vi "cluster_append.vi"(4 "Trigger line":i32, 6 "Rotary encoder":dbl, 8 "Input Cluster":T1={"Magnitude meas."=[], "Phase meas."=[], "Shift meas."=[], "cw"=TRUE, "projections per image"=0, "ramp-up readouts"=0, "current sense type"="", "Number of pulses per image"=0, "Rotation enabled"=TRUE, "Rotary position"=[], "Baseline magnitude"=0.0, "Baseline phase"=0.0, "Wait readouts"=0, "Shift waveform type"="", "Shift enabled"=TRUE, "Time domain data"=[], "Motor pulse duration"=0.0, "Shift start"=0.0, "Shift stop"=0.0, "Notes"="", "Reconstructed image"=bytes[0], "Rotary encoder type"="", "Image start"=timestamp(0 s since 1904-01-01), "Image stop"=timestamp(0 s since 1904-01-01), "readouts per projection"=0, "Recon enabled"=FALSE, "Bidirectional shift"=FALSE, "Imager mode"="", "Shift delay"=0.0, "Shift frequency"=0.0, "Image time (calc)"=0.0, "Initial encoder position"=0.0, "Recon data"=[], "Trigger line values"=[], "Bed position"=0.0, "Sample image"=bytes[0], "Patch amplitude"=0.0, "Patch frequency"=0.0, "Patch phase"=0.0}, 9 "shift value":dbl, 10 "phase value":dbl, 11 "magnitude value":dbl) -> (0 "Output Cluster":T1={"Magnitude meas."=[], "Phase meas."=[], "Shift meas."=[], "cw"=TRUE, "projections per image"=0, "ramp-up readouts"=0, "current sense type"="", "Number of pulses per image"=0, "Rotation enabled"=TRUE, "Rotary position"=[], "Baseline magnitude"=0.0, "Baseline phase"=0.0, "Wait readouts"=0, "Shift waveform type"="", "Shift enabled"=TRUE, "Time domain data"=[], "Motor pulse duration"=0.0, "Shift start"=0.0, "Shift stop"=0.0, "Notes"="", "Reconstructed image"=bytes[0], "Rotary encoder type"="", "Image start"=timestamp(0 s since 1904-01-01), "Image stop"=timestamp(0 s since 1904-01-01), "readouts per projection"=0, "Recon enabled"=FALSE, "Bidirectional shift"=FALSE, "Imager mode"="", "Shift delay"=0.0, "Shift frequency"=0.0, "Image time (calc)"=0.0, "Initial encoder position"=0.0, "Recon data"=[], "Trigger line values"=[], "Bed position"=0.0, "Sample image"=bytes[0], "Patch amplitude"=0.0, "Patch frequency"=0.0, "Patch phase"=0.0})   [LabVIEW 2019]
panel:
  # "Append Values to Cluster arrays"
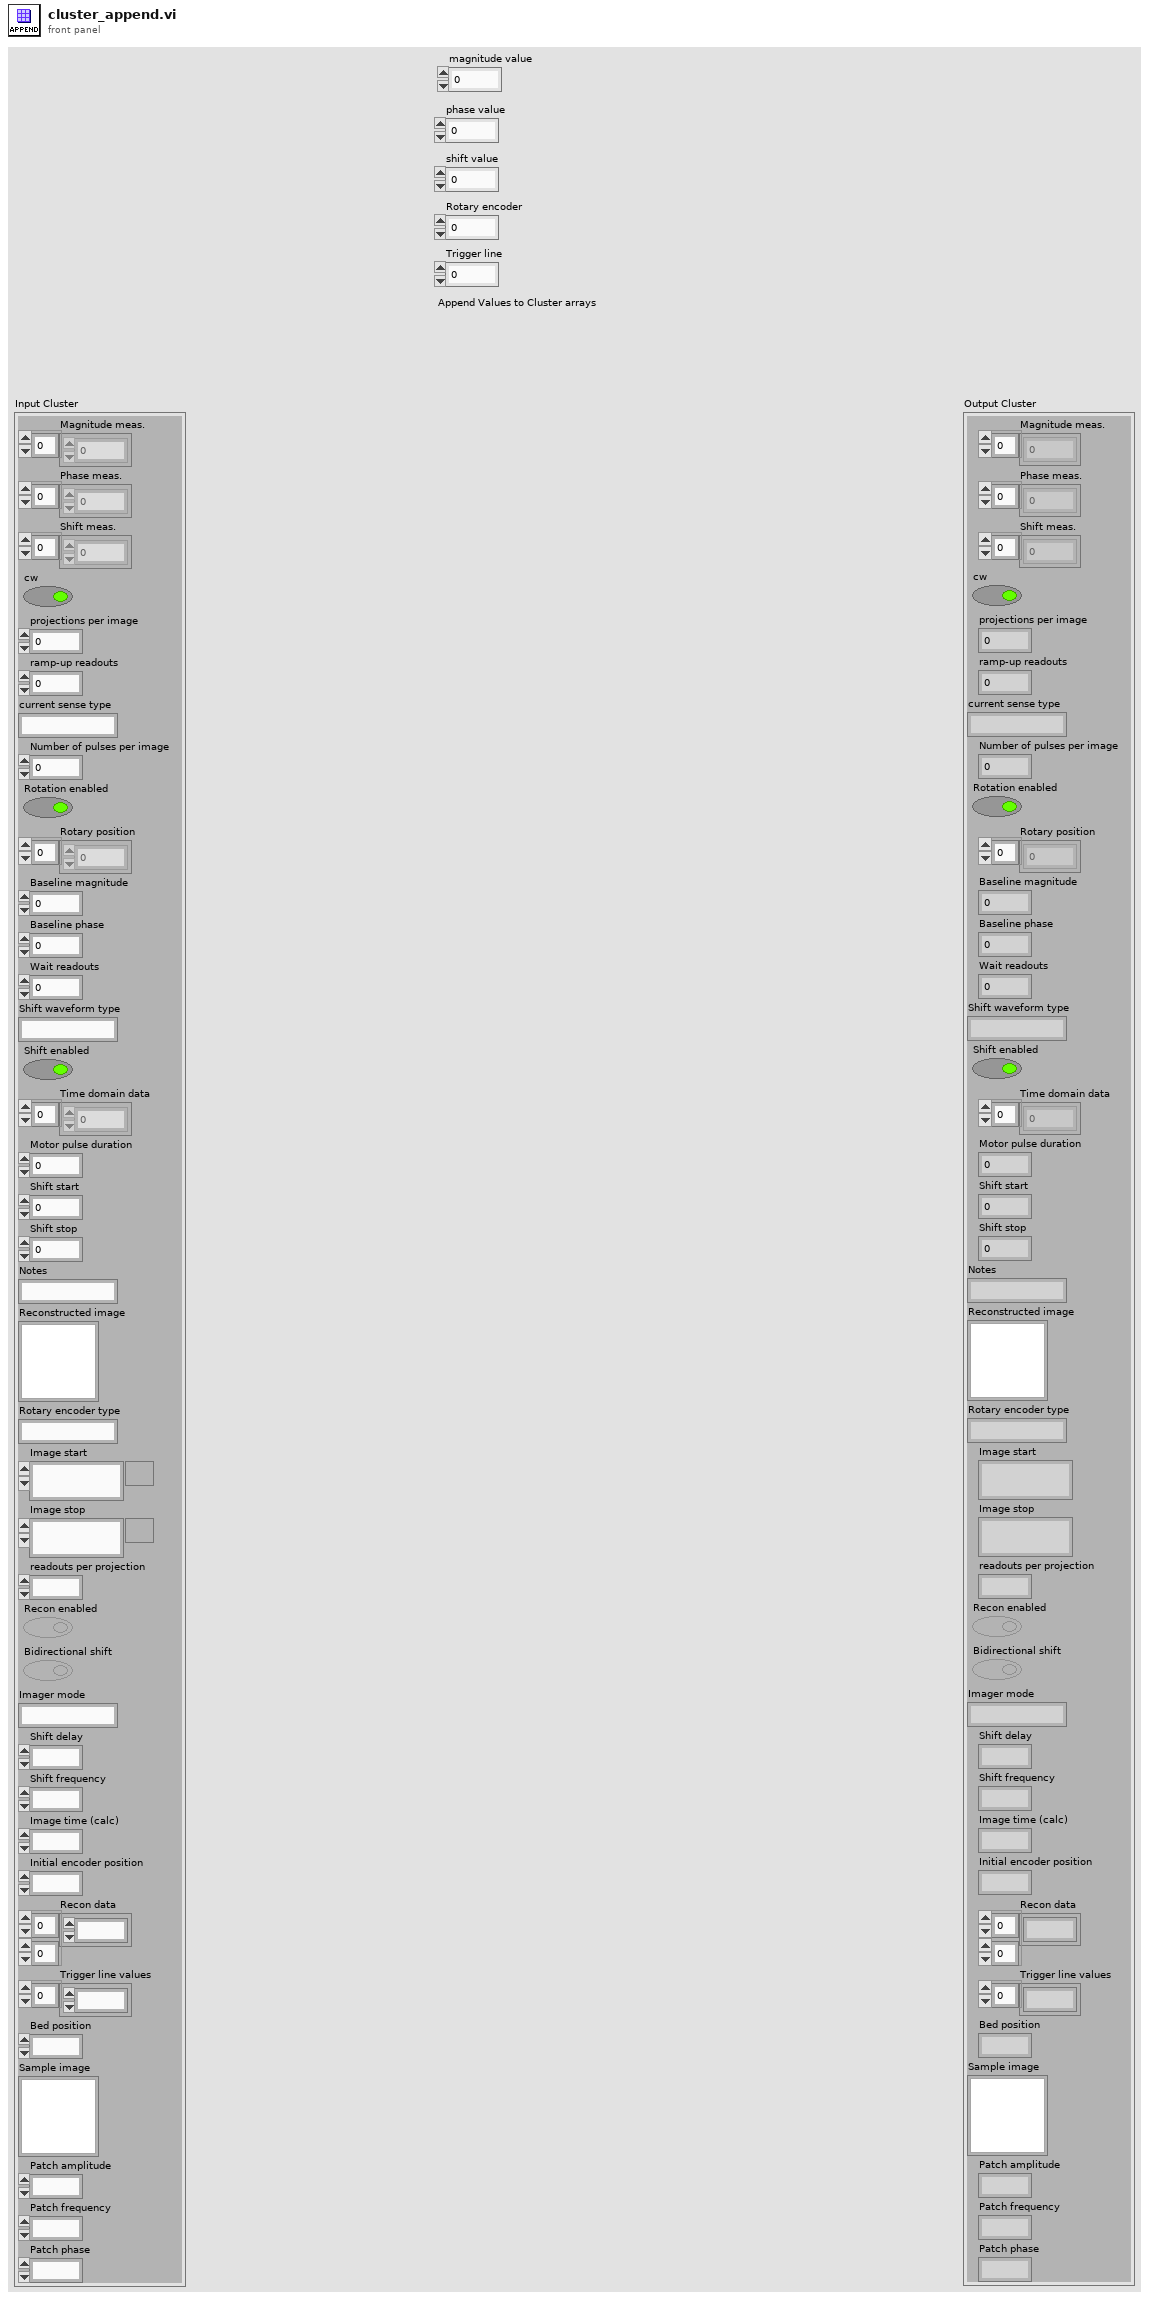
[diagram p1: front panel]
types:
  T1 = cluster{"Magnitude meas.":dbl[], "Phase meas.":dbl[], "Shift meas.":dbl[], "cw":bool, "projections per image":i32, "ramp-up readouts":i32, "current sense type":string, "Number of pulses per image":i32, "Rotation enabled":bool, "Rotary position":dbl[], "Baseline magnitude":dbl, "Baseline phase":dbl, "Wait readouts":i32, "Shift waveform type":string, "Shift enabled":bool, "Time domain data":dbl[], "Motor pulse duration":dbl, "Shift start":dbl, "Shift stop":dbl, "Notes":string, "Reconstructed image":picture, "Rotary encoder type":string, "Image start":timestamp, "Image stop":timestamp, "readouts per projection":i32, "Recon enabled":bool, "Bidirectional shift":bool, "Imager mode":string, "Shift delay":dbl, "Shift frequency":dbl, "Image time (calc)":dbl, "Initial encoder position":dbl, "Recon data":dbl[][], "Trigger line values":i32[], "Bed position":dbl, "Sample image":picture, "Patch amplitude":dbl, "Patch frequency":dbl, "Patch phase":dbl}
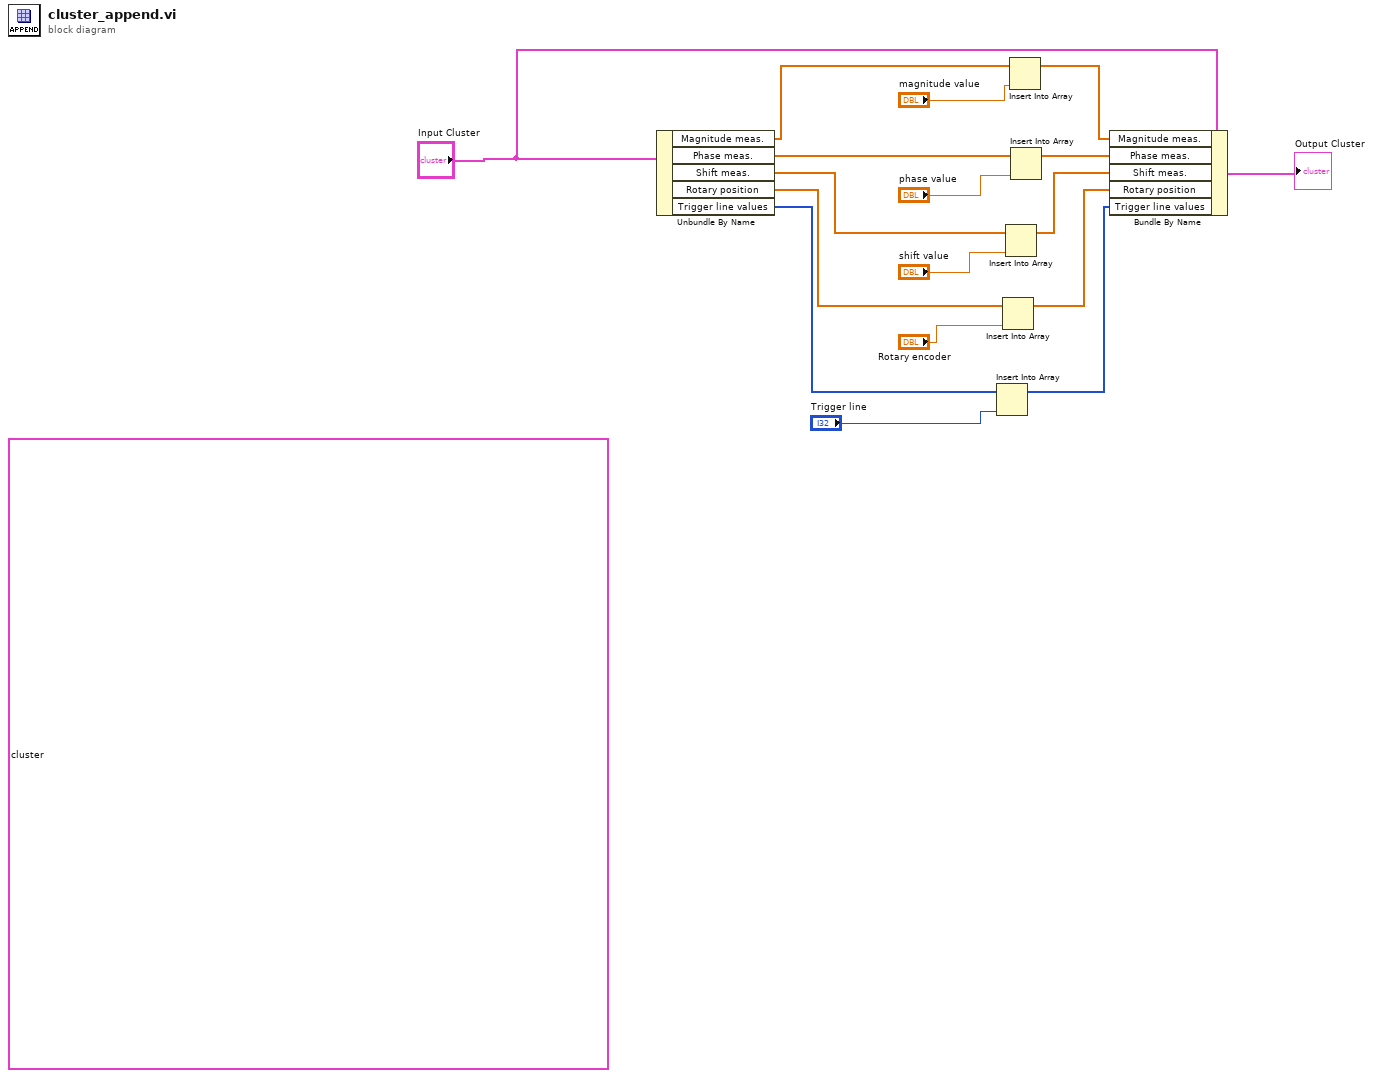
[diagram p0: block diagram]
diagram:
  (unwired) T1 {"Magnitude meas."=[], "Phase meas."=[], "Shift meas."=[], "cw"=TRUE, "projections per image"=0, "ramp-up readouts"=0, "current sense type"="", "Number of pulses per image"=0, "Rotation enabled"=TRUE, "Rotary position"=[], "Baseline magnitude"=0.0, "Baseline phase"=0.0, "Wait readouts"=0, "Shift waveform type"="", "Shift enabled"=TRUE, "Time domain data"=[], "Motor pulse duration"=0.0, "Shift start"=0.0, "Shift stop"=0.0, "Notes"="", "Reconstructed image"=bytes[0], "Rotary encoder type"="", "Image start"=timestamp(0 s since 1904-01-01), "Image stop"=timestamp(0 s since 1904-01-01), "readouts per projection"=0, "Recon enabled"=FALSE, "Bidirectional shift"=FALSE, "Imager mode"="", "Shift delay"=0.0, "Shift frequency"=0.0, "Image time (calc)"=0.0, "Initial encoder position"=0.0, "Recon data"=[], "Trigger line values"=[], "Bed position"=0.0, "Sample image"=bytes[0], "Patch amplitude"=0.0, "Patch frequency"=0.0, "Patch phase"=0.0}
  n1 = Unbundle By Name("Input Cluster") -> ("Magnitude meas."=w12:dbl[], "Phase meas."=w15:dbl[], "Shift meas."=w13:dbl[], "Rotary position"=w7:dbl[], "Trigger line values"=w5:i32[])
  n2 = Insert Into Array(array=w5, new element="Trigger line") -> (w3:i32[])  [unwired: 1 in]
  n3 = Insert Into Array(array=w7, new element="Rotary encoder") -> (w8:dbl[])  [unwired: 1 in]
  n4 = Insert Into Array(array=w13, new element="shift value") -> (w9:dbl[])  [unwired: 1 in]
  n5 = Insert Into Array(array=w12, new element="magnitude value") -> (w11:dbl[])  [unwired: 1 in]
  n6 = Insert Into Array(array=w15, new element="phase value") -> (w10:dbl[])  [unwired: 1 in]
  n7 = Bundle By Name(cluster="Input Cluster", "Magnitude meas."=w11, "Phase meas."=w10, "Shift meas."=w9, "Rotary position"=w8, "Trigger line values"=w3) -> (→"Output Cluster":T1)
